vi "Test CONNECT packet.vi"(8 "error in (no error)":errorcluster) -> (0 "error out":errorcluster)   [LabVIEW 2013]
uses:
  source/Control Packets/CONNECT/CONNECT.lvclass
  source/Control Packets/CONNECT/ConnectFlags -- cluster.ctl
  source/Control Packets/ControlPacket/ControlPacket.lvclass
  <vilib>/addons/_JKI Toolkits/Caraya/classes/Test/Test.lvclass
  <vilib>/addons/_JKI Toolkits/Caraya/classes/Assert/Assert.lvclass
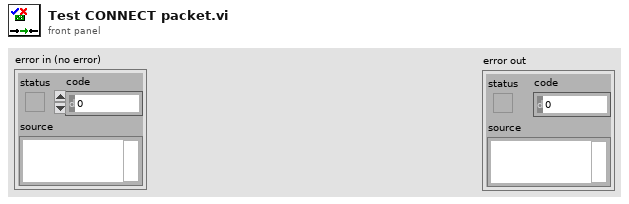
[diagram p1: front panel]
types:
  T1 = cluster{"Will Topic":string, "Will Message":string, "Username":string, "Password":string}
  T2 = typedef "CONNECT.lvclass/ConnectFlags -- cluster.ctl" = cluster{"Reserved":bool, "Clean Session":bool, "Will Flag":bool, "Will QoS 1":bool, "Will QoS 2":bool, "Will Retain":bool, "Password Flag":bool, "User Name Flag":bool}
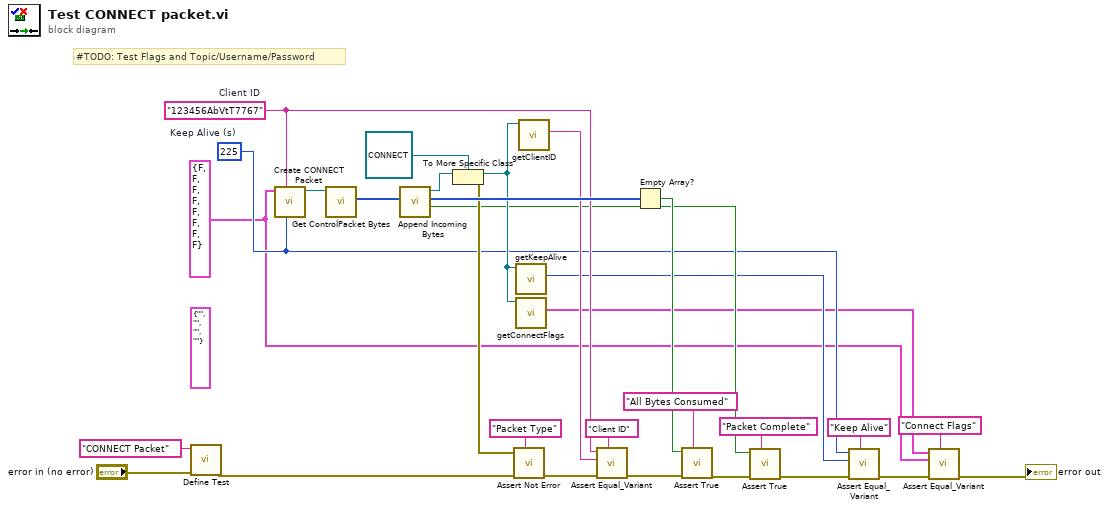
[diagram p0: block diagram]
diagram:
  (unwired) T1 {"Will Topic"="", "Will Message"="", "Username"="", "Password"=""} ("Payload")
  w1 = T2 {"Reserved"=FALSE, "Clean Session"=FALSE, "Will Flag"=FALSE, "Will QoS 1"=FALSE, "Will QoS 2"=FALSE, "Will Retain"=FALSE, "Password Flag"=FALSE, "User Name Flag"=FALSE} ("Connect Flags")
  w7 = u16 225  # Keep Alive (s)
  w18 = "123456AbVtT7767"  # Client ID
  # "#TODO: Test Flags and Topic/Username/Password"
  n1 = call <vilib>:"Define Test.vi"("error in (no error)"="error in (no error)", "Label (VI Title)"="CONNECT Packet") -> ("error out"=w22:errorcluster)  [unwired: 9 in]
  n2 = call "Create CONNECT Packet.vi"("Keep Alive (s)"=w7, "Client ID (empty: generate new)"=w18, "Connect Flags"=w1) -> ("CONNECT"=w30:refnum<class "CONNECT.lvclass">)  [unwired: 7 in, 1 out]
  n3 = call "Get ControlPacket Bytes.vi"("ControlPacket"=w30) -> ("Bytes Stream"=w29:u8[])  [unwired: 8 in, 2 out]
  n4 = call "Append Incoming Bytes.vi"("Incoming Packets"=w29) -> ("Complete Packet"=w11:bool, "Remaining Packets"=w28:u8[], "ControlPacket"=w27:refnum<class "ControlPacket.lvclass">)  [unwired: 7 in, 1 out]
  n5 = To More Specific Class(target class=refnum<class "CONNECT.lvclass"> refnum ("CONNECT in"), reference=w27) -> (specific class reference=w25:refnum<class "CONNECT.lvclass">, error out=w21:errorcluster)  [unwired: 1 in]
  n6 = call <vilib>:"Assert Not Error.vi"("Label"="Packet Type" ("Label (VI Title)"), "error in (no error)"=w22, "Not Error?"=w21) -> ("error out"=w19:errorcluster)  [unwired: 8 in]
  n7 = call "getKeepAlive.vi"("CONNECT in"=w25) -> ("Keep Alive (s)"=w6:u16)  [unwired: 9 in, 1 out]
  n8 = call "getConnectFlags.vi"("CONNECT in"=w25) -> ("Connect Flags"=w2:T2)  [unwired: 9 in, 1 out]
  n9 = call "getClientID.vi"("CONNECT in"=w25) -> ("Client ID"=w17:string)  [unwired: 9 in, 1 out]
  n10 = call <vilib>:"Assert Equal_Variant.vi"("Label"="Client ID" ("Label (VI Title)"), "error in (no error)"=w19, "Y"=w17, "X"=w18) -> ("error out"=w15:errorcluster)  [unwired: 7 in]
  n11 = Empty Array?(array=w28) -> (empty?=w14:bool)
  n12 = call <vilib>:"Assert True.vi"("Label"="All Bytes Consumed" ("Label (VI Title)"), "error in (no error)"=w15, "True?"=w14) -> ("error out"=w12:errorcluster)  [unwired: 8 in]
  n13 = call <vilib>:"Assert True.vi"("Label"="Packet Complete" ("Label (VI Title)"), "error in (no error)"=w12, "True?"=w11) -> ("error out"=w8:errorcluster)  [unwired: 8 in]
  n14 = call <vilib>:"Assert Equal_Variant.vi"("Label"="Keep Alive" ("Label (VI Title)"), "error in (no error)"=w8, "Y"=w6, "X"=w7) -> ("error out"=w4:errorcluster)  [unwired: 7 in]
  n15 = call <vilib>:"Assert Equal_Variant.vi"("Label"="Connect Flags" ("Label (VI Title)"), "error in (no error)"=w4, "Y"=w1, "X"=w2) -> ("error out"=→"error out":errorcluster)  [unwired: 7 in]
